vi "TP_OP_Queue.vi"(6 "max queue size (-1, unlimited)":i32=-1, 7 "OP_Queue (get queue)":T1(ring)=enum."Get Queue", 8 "error in":errorcluster, 11 "name (unnamed)":string) -> (0 "error out":errorcluster, 3 "queue out":refnum<queue>)   [LabVIEW 2012]
uses:
  support/Message Queue/Message Cluster.ctl
  support/Message Queue/TP_Message Queue.lvlib
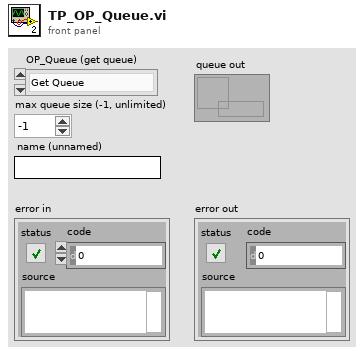
[diagram p1: front panel]
types:
  T1 = enum16{"Create Queue", "Get Queue", "Destory Queue"}
  T2 = typedef "TP_Message Queue.lvlib/Message Cluster.ctl" = cluster{"Message":string, "Message Data":variant}
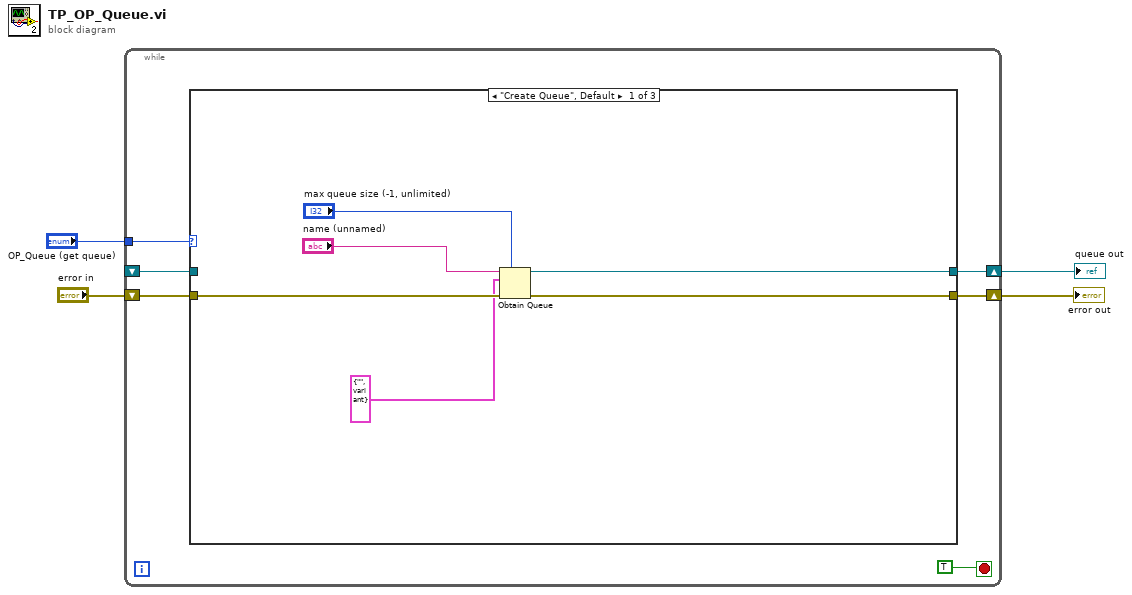
[diagram p0: block diagram]
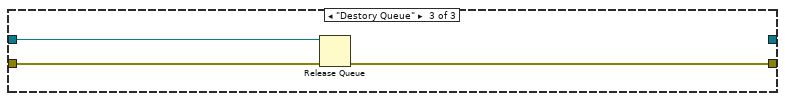
[diagram p3: hidden frame]
diagram:
  n1 = while {
    tunnel: "OP_Queue (get queue)" -> [w9]
    shift-right: [w8] -> w1
    shift-left: _ -> [w7]
    shift-right: [w5] -> w3
    shift-left: "error in" -> [w6]
    stop <- TRUE stop-if-true
    n2 = case shown="\"Create Queue\", Default" w9 {
      tunnel: [w16 w18 _] -> w8
      tunnel: w7 -> [_ w18 w19]
      tunnel: w6 -> [w13 w17 w21]
      tunnel: [w12 w17 w20] -> w5
      frame "Create Queue", Default {
        n3 = Obtain Queue(max queue size (-1, unlimited)="max queue size (-1, unlimited)", name (unnamed)="name (unnamed)", element data type=T2 {"Message"="", "Message Data"=variant} ("Message Cluster"), error in (no error)=w13) -> (queue out=w16:refnum<queue>, error out=w12:errorcluster)  [unwired: 1 in, 1 out]
      }
      frame "Get Queue" {
      }
      frame "Destory Queue" {
        n4 = Release Queue(queue=w19, error in (no error)=w21) -> (error out=w20:errorcluster)  [unwired: 1 in, 2 out]
      }
    }
  }
  "error out" <- w3
  "queue out" <- w1
